vi "Check All Caliper Steps.vi"(9 "Analysis_Point_Result":T1[](array[typedef]), 11 "CaliperEntryList":T2[](array[typedef]) {"CaliperType" items=["Distance", "Mid Point", "Perpendicular Projection", "Lines Intersection", "Angle from Horizontal", "Angle from Vertical", "Angle Defined by 3 Points", "Angle Defined by 4 Points", "Bissecting Line", "Mid Line", "Center of Mass", "Area", "Line Fit", "Circle Fit", "Ellipse Fit"]}) -> (0 "error out":errorcluster, 2 "Index":i32, 3 "CaliperEntryOut":T2[](array[typedef]) {"CaliperType" items=["Distance", "Mid Point", "Perpendicular Projection", "Lines Intersection", "Angle from Horizontal", "Angle from Vertical", "Angle Defined by 3 Points", "Angle Defined by 4 Points", "Bissecting Line", "Mid Line", "Center of Mass", "Area", "Line Fit", "Circle Fit", "Ellipse Fit"]})   [LabVIEW 2019]
uses:
  Controls/CaliperDataEntry.ctl
  Controls/CaliperType.ctl
  Controls/SelectionListEntry.ctl
  Controls/SelectionListEntryPointType.ctl
  Controls/CaliperResult.ctl
  Analysis/Controls/Analysis_Result_To_Caliper.ctl
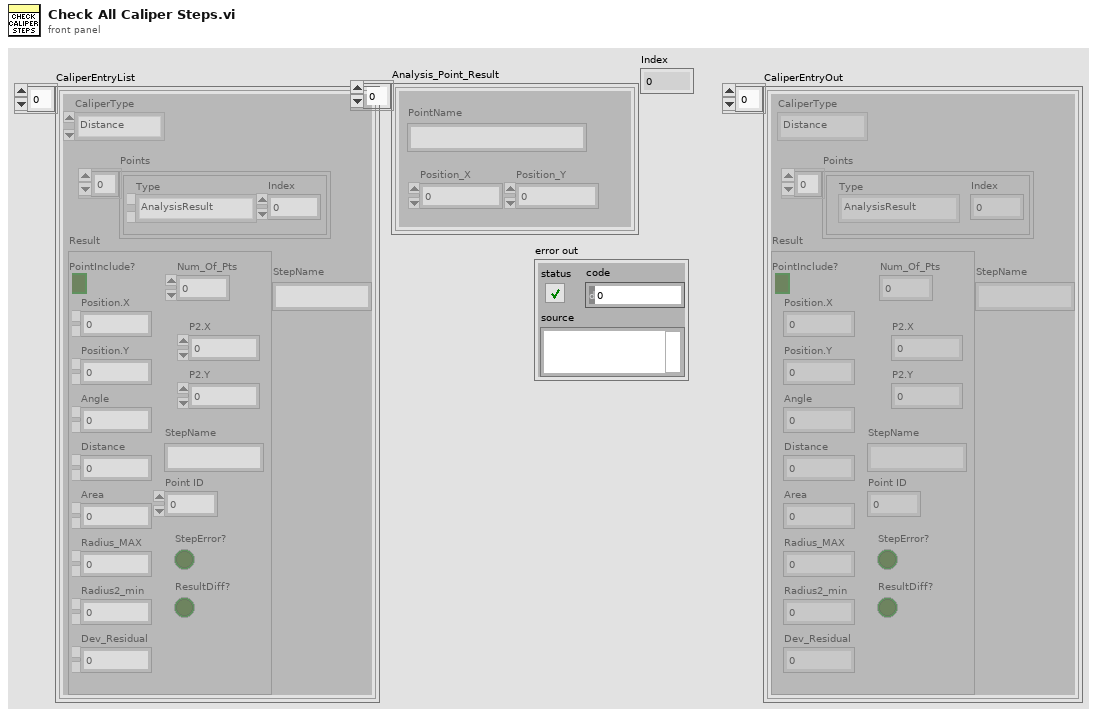
[diagram p1: front panel]
types:
  T1 = typedef "Analysis_Result_To_Caliper.ctl" = cluster{"PointName":string, "Position_X":dbl, "Position_Y":dbl}
  T2 = typedef "CaliperDataEntry.ctl" = cluster{"CaliperType":T3, "Points":T4[], "Result":T6, "StepName":string}
  T3 = typedef "CaliperType.ctl" = u32
  T4 = typedef "SelectionListEntry.ctl" = cluster{"Type":T5, "Index":i32}
  T5 = typedef "SelectionListEntryPointType.ctl" = enum16{"AnalysisResult", "CaliperResult"}
  T6 = typedef "CaliperResult.ctl" = cluster{"PointInclude?":bool, "Num_Of_Pts":u8, "Position.X":dbl, "Position.Y":dbl, "Angle":dbl, "Distance":dbl, "Area":dbl, "Radius_MAX":dbl, "Radius2_min":dbl, "Dev_Residual":dbl, "P2.X":dbl, "P2.Y":dbl, "StepName":string, "Point ID":u8, "StepError?":bool, "ResultDiff?":bool}
  T7 = typedef "CaliperDataEntry_SinglePoint.ctl" = cluster{"CaliperType":T3, "Points":T4[], "Result":T8, "StepName":string}
  T8 = typedef "CaliperResult_SinglePoint.ctl" = cluster{"PointInclude?":bool, "Position.X":dbl, "Position.Y":dbl, "Angle":dbl, "Distance":dbl, "Area":dbl, "Radius_MAX":dbl, "Radius2_min":dbl, "Dev_Residual":dbl, "StepName":string, "Point ID":u8, "StepError?":bool, "ResultDiff?":bool}
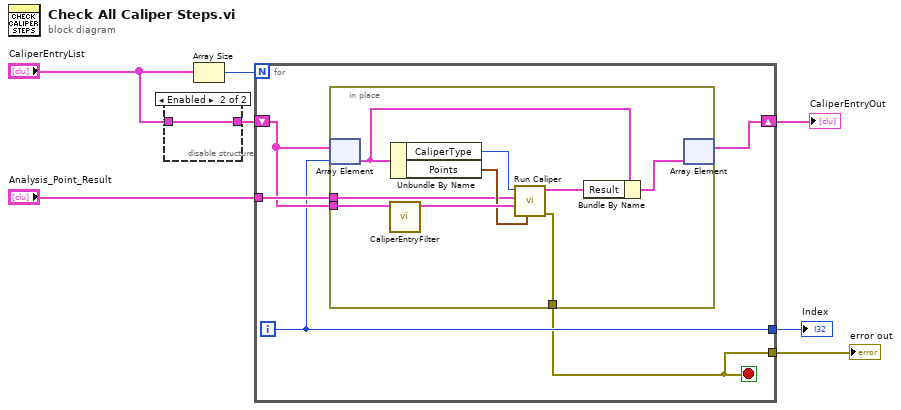
[diagram p0: block diagram]
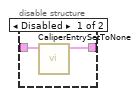
[diagram p2: hidden frame]
diagram:
  n1 = disable-structure shown="Enabled" {
    disable-tunnel: [w9 w10] -> w6
    disable-tunnel: "CaliperEntryList" -> [w8 w10]
    frame Disabled {
      n2 = call "CaliperEntrySetToNone.vi"("CaliperEntryList"=w8) -> ("CaliperEntryOut"=w9:T2[])  [unwired: 9 in, 1 out]
    }
    frame Enabled {
    }
  }
  n3 = Array Size(array="CaliperEntryList") -> (size(s)=w7:i32)
  n4 = for {
    N: w7 -> [_]
    tunnel: "Analysis_Point_Result" -> [w15]
    shift-right: [w13] -> w4
    shift-left: w6 -> [w14]
    tunnel: [w12] -> w1
    tunnel: [w11] -> w2
    i -> [w12]
    stop <- w11 stop-if-true
    n5 = in-place {
      in-place-border: w15 -> [w21]
      in-place-border: w14 -> [w20]
      in-place-border: [w16] -> w11
      n6 = in-place-array #1(w14, w12) -> (w19:T2)
      n7 = call "CaliperEntryFilter.vi"("CaliperEntryList"=w20) -> ("FilteredCaliperEntry"=w24:T7[])  [unwired: 10 in]
      n8 = Unbundle By Name(w19) -> ("CaliperType"=w23:T3, "Points"=w22:T4[])
      n9 = call "Run Caliper.vi"("SelectionList"=w22, "FilteredCaliperEntry"=w24, "Analysis_Point_Result"=w21, "CaliperType"=w23) -> ("error out"=w16:errorcluster, "Result"=w17:T6)  [unwired: 5 in, 1 out]
      n10 = Bundle By Name(cluster=w19, "Result"=w17) -> (w18:T2)
      n11 = in-place-array #1(w18) -> (w13:T2[])  [unwired: 1 out]
    }
  }
  "CaliperEntryOut" <- w4
  "error out" <- w2
  "Index" <- w1
